vi "bigcryo_Harry-RH - step v1.vi"(6 "Mag Field Step":dbl=0.002, 7 "Directory Output":string="C:\\User Data\\hlb54\\210111_42B\\JJ1\\IcH_pos_to_neg_T=4p00K_set=0p0T", 8 "Stop Field":dbl=-0.2, 9 "Start Field (T)":dbl=0.2 format="%#_7f", 10 "Stop":bool, 11 "Measure":bool) -> ()   [LabVIEW 2019]
uses:
  Global 2.vi
  B_Globals.vi
  <vilib>/Utility/file.llb/Read From Spreadsheet File (DBL).vi
panel:
  out "B [T]":dbl
  out "Sample Temp [K] - Meas":dbl=1.55928
  out "I - Count":cluster{i32[], dbl[]}(graph) caption="XY Graph"
  out "Status":string="Welcome!"
  in  "Keithley":refnum<visa-resource-name>="GPIB1::20::INSTR"
  in  "Delay [sec]":dbl=0.002 format="%#_6e"
  in  "Compliance [V] 2":dbl=10.0 format="%#_6f"
  in  "Abort Conductance":bool
  in  "Count [A]":dbl=1e-05 format="%#_6e"
  in  "I-Max [A]":dbl=0.002 format="%#_6e"
  in  "Arm Conductance":bool
  in  "Minicryo":bool=TRUE
  in  "Field and rate":dbl[][](array[numeric])
  in  "step":bool=TRUE
  in  "Set Rate (T/min)":dbl=0.1
  out "Iteration?":i32=401
  out "B Aim":dbl=-0.202
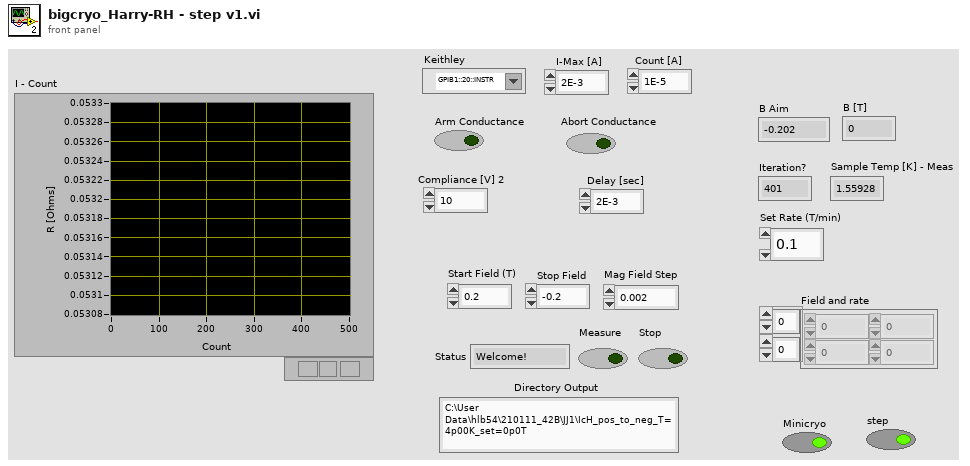
[diagram p1: front panel]
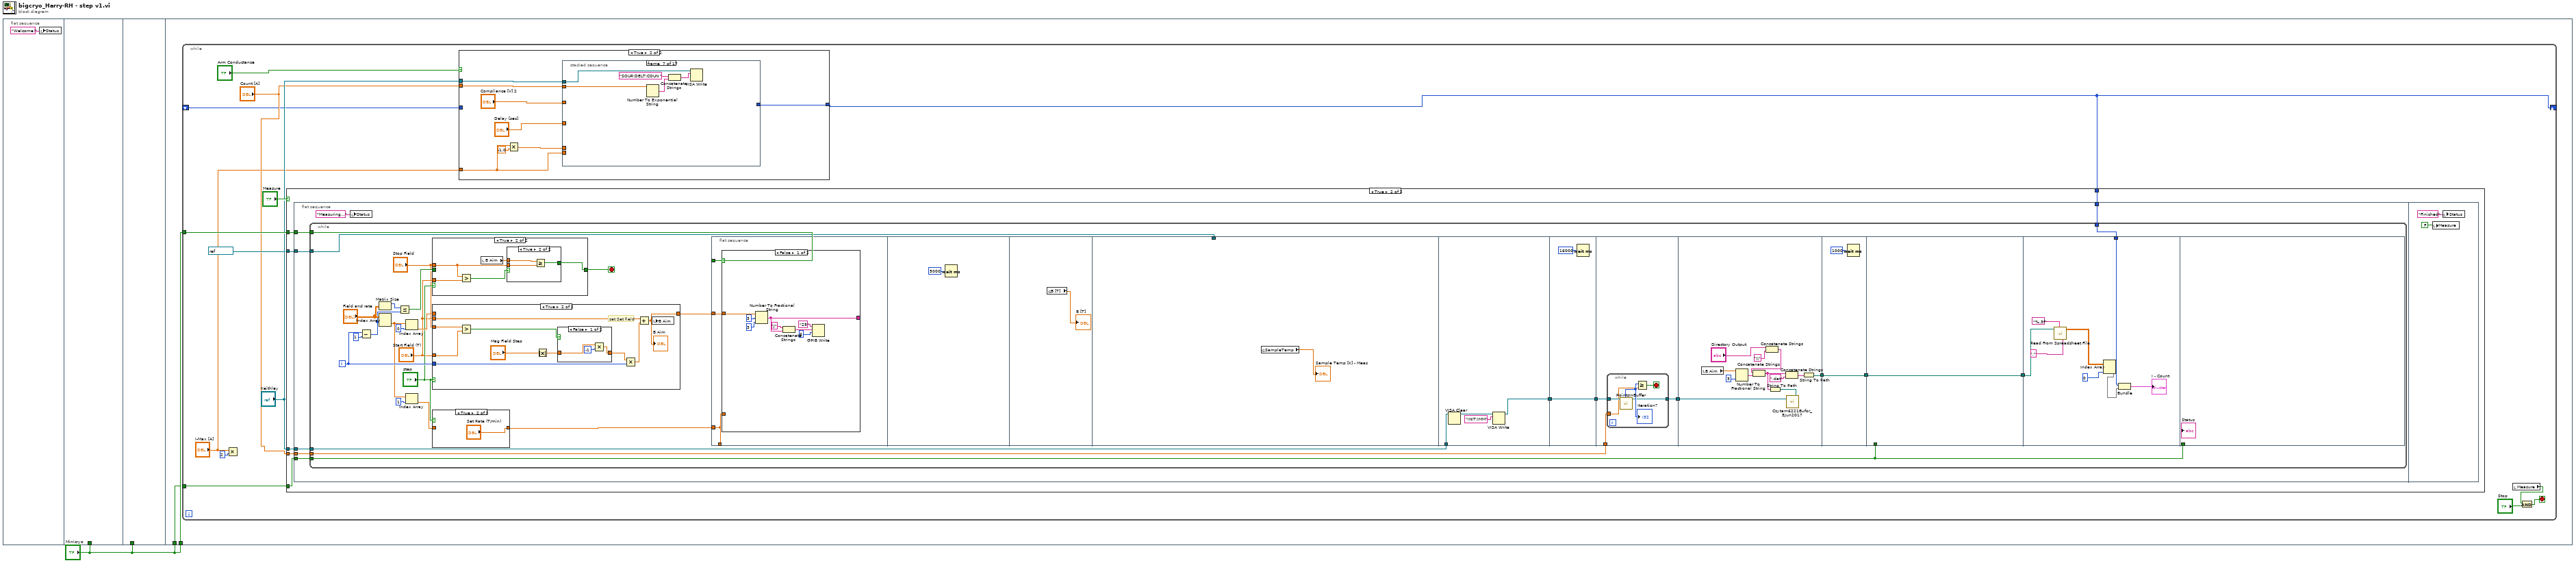
[diagram p0: block diagram]
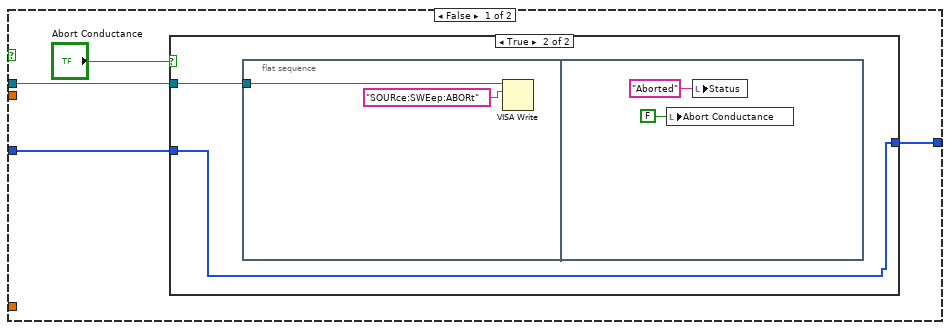
[diagram p2: hidden frame]
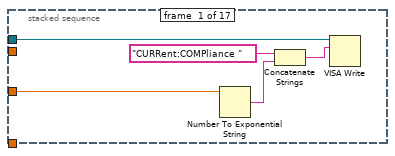
[diagram p4: hidden frame]
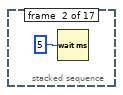
[diagram p5: hidden frame]
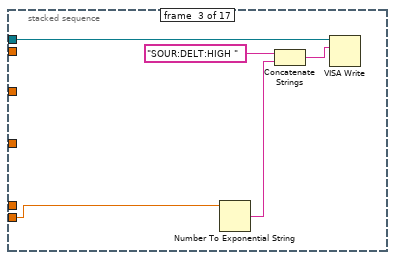
[diagram p6: hidden frame]
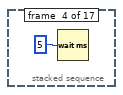
[diagram p7: hidden frame]
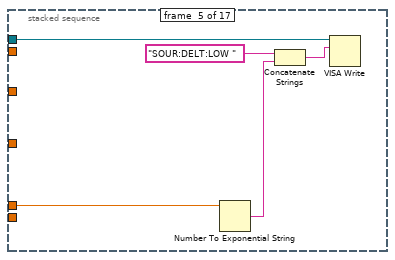
[diagram p8: hidden frame]
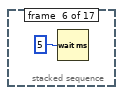
[diagram p9: hidden frame]
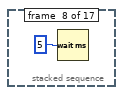
[diagram p10: hidden frame]
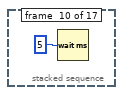
[diagram p12: hidden frame]
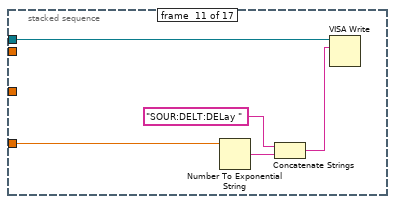
[diagram p13: hidden frame]
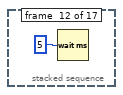
[diagram p14: hidden frame]
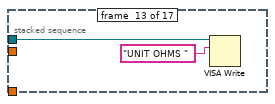
[diagram p15: hidden frame]
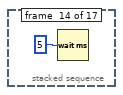
[diagram p16: hidden frame]
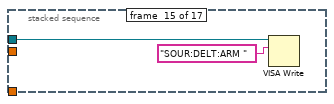
[diagram p17: hidden frame]
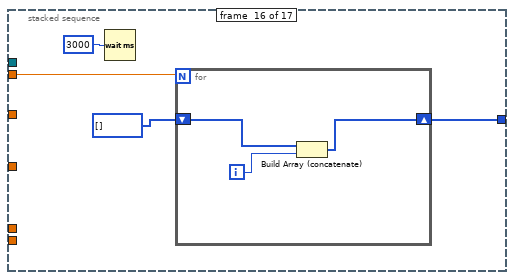
[diagram p18: hidden frame]
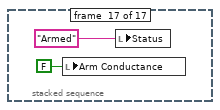
[diagram p19: hidden frame]
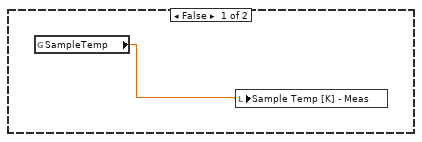
[diagram p20: hidden frame]
diagram:
  n1 = flat-sequence {
    tunnel: "Minicryo" -> [_]
    tunnel: "Minicryo" -> [_]
    tunnel: "Minicryo" -> [w4]
    tunnel: "Minicryo" -> [w3]
    frame #0 {
      n2 = local write "Status"("Welcome!") -> ()
    }
    frame #1 {
    }
    frame #2 {
    }
    frame #3 {
      n3 = while {
        tunnel: w4 -> [w18]
        tunnel: w3 -> [w17]
        shift-right: [w5] -> _
        shift-left: _ -> [w6]
        stop <- w9 stop-if-true
        n4 = Multiply(x="I-Max [A]", y=2) -> ()  [unwired: 1 out]
        n5 = case shown="True" "Arm Conductance" {
          tunnel: "Keithley" -> [w21 w34]
          tunnel: "Count [A]" -> [_ w33]
          tunnel: "I-Max [A]" -> [_ w31]
          tunnel: [w19 w30] -> w5
          tunnel: w6 -> [w20 _]
          frame False {
            n6 = case shown="True" "Abort Conductance" {
              tunnel: w21 -> [_ w25]
              tunnel: w20 -> [w23 w24]
              tunnel: [w23 w24] -> w19
              frame False {
              }
              frame True {
                n7 = flat-sequence {
                  tunnel: w25 -> [w26]
                  frame #0 {
                    n8 = VISA Write(VISA resource name=w26, write buffer="SOURce:SWEep:ABORt") -> ()  [unwired: 1 in, 3 out]
                  }
                  frame #1 {
                    n9 = local write "Abort Conductance"(FALSE) -> ()
                    n10 = local write "Status"("Aborted") -> ()
                  }
                }
              }
            }
          }
          frame True {
            n11 = Multiply(x=w31, y=-1.0) -> (x*y=w32:dbl)
            n12 = stacked-sequence {
              tunnel: w32 -> [_ _ _ _ w50 _ _ _ _ _ _ _ _ _ _ _ _]
              tunnel: "Delay [sec]" -> [_ _ _ _ _ _ _ _ _ _ w64 _ _ _ _ _ _]
              tunnel: "Compliance [V] 2" -> [w39 _ _ _ _ _ _ _ _ _ _ _ _ _ _ _ _]
              tunnel: w34 -> [w38 _ w45 _ w51 _ w57 _ _ _ w63 _ w69 _ w72 _ _]
              tunnel: w33 -> [_ _ _ _ _ _ w56 _ _ _ _ _ _ _ _ w74 _]
              tunnel: w31 -> [_ _ w44 _ _ _ _ _ _ _ _ _ _ _ _ _ _]
              tunnel: [_ _ _ _ _ _ _ _ _ _ _ _ _ _ _ w75 _] -> w30
              frame #0 {
                n13 = Number To Exponential String(number=w39) -> (E-format string=w41:string)  [unwired: 3 in]
                n14 = Concatenate Strings("CURRent:COMPliance ", w41) -> (w40:string)
                n15 = VISA Write(VISA resource name=w38, write buffer=w40) -> ()  [unwired: 1 in, 3 out]
              }
              frame #1 {
                n16 = Wait (ms)(milliseconds to wait=5) -> ()  [unwired: 1 out]
              }
              frame #2 {
                n17 = Number To Exponential String(number=w44) -> (E-format string=w47:string)  [unwired: 3 in]
                n18 = Concatenate Strings("SOUR:DELT:HIGH ", w47) -> (w46:string)
                n19 = VISA Write(VISA resource name=w45, write buffer=w46) -> ()  [unwired: 1 in, 3 out]
              }
              frame #3 {
                n20 = Wait (ms)(milliseconds to wait=5) -> ()  [unwired: 1 out]
              }
              frame #4 {
                n21 = Number To Exponential String(number=w50) -> (E-format string=w53:string)  [unwired: 3 in]
                n22 = Concatenate Strings("SOUR:DELT:LOW ", w53) -> (w52:string)
                n23 = VISA Write(VISA resource name=w51, write buffer=w52) -> ()  [unwired: 1 in, 3 out]
              }
              frame #5 {
                n24 = Wait (ms)(milliseconds to wait=5) -> ()  [unwired: 1 out]
              }
              frame #6 {
                n25 = Number To Exponential String(number=w56) -> (E-format string=w59:string)  [unwired: 3 in]
                n26 = Concatenate Strings("SOUR:DELT:COUN ", w59) -> (w58:string)
                n27 = VISA Write(VISA resource name=w57, write buffer=w58) -> ()  [unwired: 1 in, 3 out]
              }
              frame #7 {
                n28 = Wait (ms)(milliseconds to wait=5) -> ()  [unwired: 1 out]
              }
              frame #8 {
              }
              frame #9 {
                n29 = Wait (ms)(milliseconds to wait=5) -> ()  [unwired: 1 out]
              }
              frame #10 {
                n30 = Number To Exponential String(number=w64) -> (E-format string=w66:string)  [unwired: 3 in]
                n31 = Concatenate Strings("SOUR:DELT:DELay ", w66) -> (w65:string)
                n32 = VISA Write(VISA resource name=w63, write buffer=w65) -> ()  [unwired: 1 in, 3 out]
              }
              frame #11 {
                n33 = Wait (ms)(milliseconds to wait=5) -> ()  [unwired: 1 out]
              }
              frame #12 {
                n34 = VISA Write(VISA resource name=w69, write buffer="UNIT OHMS ") -> ()  [unwired: 1 in, 3 out]
              }
              frame #13 {
                n35 = Wait (ms)(milliseconds to wait=5) -> ()  [unwired: 1 out]
              }
              frame #14 {
                n36 = VISA Write(VISA resource name=w72, write buffer="SOUR:DELT:ARM ") -> ()  [unwired: 1 in, 3 out]
              }
              frame #15 {
                n37 = Wait (ms)(milliseconds to wait=3000) -> ()  [unwired: 1 out]
                n38 = for {
                  N: w74 -> [_]
                  shift-right: [w79] -> w75
                  shift-left: i32[] [] -> [w80]
                  i -> [w78]
                  n39 = Build Array (concatenate)(w80, w78) -> (w79:i32[])
                }
              }
              frame #16 {
                n40 = local write "Arm Conductance"(FALSE) -> ()
                n41 = local write "Status"("Armed") -> ()
              }
            }
          }
        }
        n42 = case shown="True" "Measure" {
          tunnel: w18 -> [_ w89]
          tunnel: w17 -> [_ w88]
          tunnel: "Keithley" -> [_ w87]
          tunnel: "Count [A]" -> [_ w86]
          tunnel: refnum<visa-resource-name> "COM7" ("LakeShore340") -> [_ w85]
          tunnel: w5 -> [_ w84]
          frame False {
            n43 = global read "Global 2.vi" "SampleTemp"() -> (w83:dbl)
            n44 = local write "Sample Temp [K] - Meas"(w83) -> ()
          }
          frame True {
            n45 = flat-sequence {
              tunnel: w89 -> [w96]
              tunnel: w88 -> [w95]
              tunnel: w87 -> [w94]
              tunnel: w86 -> [w93]
              tunnel: w85 -> [w91]
              tunnel: w84 -> [w90]
              frame #0 {
                n46 = while {
                  tunnel: w96 -> [w113]
                  tunnel: w95 -> [w108]
                  tunnel: w94 -> [w106]
                  tunnel: w93 -> [w105]
                  tunnel: w91 -> [w98]
                  tunnel: w90 -> [w97]
                  i -> [w119]
                  stop <- w104 stop-if-true
                  n47 = Subtract(x=w119, y=1) -> (x-y=w110:i32)
                  n48 = Matrix Size(0:"Field and rate") -> (1:w111:i32)  [unwired: 1 out]
                  n49 = Index Array(array="Field and rate", index (row)=w110) -> (element=w116:dbl[])  [unwired: 1 in]
                  n50 = Less Or Equal?(x=w111, y=w110) -> (x <= y?=w109:bool)
                  n51 = Index Array(array=w116, index=0) -> (element=w115:dbl)
                  n52 = Index Array(array=w116, index=1) -> (element=w114:dbl)
                  n53 = case shown="True" "step" {
                    tunnel: [w126 w131] -> w104
                    tunnel: w109 -> [w126 _]
                    tunnel: "Stop Field" -> [_ w129]
                    tunnel: "Start Field (T)" -> [_ w128]
                    frame False {
                    }
                    frame True {
                      n54 = Greater?(x=w129, y=w128) -> (0:w127:bool)
                      n55 = local read "B Aim"() -> (w130:dbl)
                      n56 = case shown="True" w127 {
                        tunnel: [w134 w137] -> w131
                        tunnel: w130 -> [w132 w136]
                        tunnel: w129 -> [w133 w135]
                        frame False {
                          n57 = Less Or Equal?(x=w132, y=w133) -> (x <= y?=w134:bool)
                        }
                        frame True {
                          n58 = Greater Or Equal?(x=w136, y=w135) -> (x >= y?=w137:bool)
                        }
                      }
                    }
                  }
                  n59 = case shown="True" "step" {
                    tunnel: [w140 w149] -> w125
                    tunnel: w119 -> [_ w148]
                    tunnel: w115 -> [w140 _]
                    tunnel: "Start Field (T)" -> [_ w147]
                    tunnel: "Start Field (T)" -> [_ w146]
                    tunnel: "Stop Field" -> [_ w145]
                    frame False {
                    }
                    frame True {
                      # "set Set field"
                      n60 = Greater?(x=w145, y=w146) -> (0:w141:bool)
                      n61 = Absolute Value(x="Mag Field Step") -> (abs(x)=w143:dbl)
                      n62 = case shown="False" w141 {
                        tunnel: [w153 w154] -> w142
                        tunnel: w143 -> [w151 w154]
                        frame False {
                          n63 = Multiply(x=w151, y=-1) -> (x*y=w153:dbl)
                        }
                        frame True {
                        }
                      }
                      n64 = Multiply(x=w142, y=w148) -> (x*y=w150:dbl)
                      n65 = Add(x=w147, y=w150) -> (x+y=w149:dbl)
                      "B Aim" <- w149
                      n66 = local write "B Aim"(w149) -> ()
                    }
                  }
                  n67 = case shown="True" "step" {
                    tunnel: [w138 "Set Rate (T/min)"] -> w121
                    tunnel: w114 -> [w138 _]
                    frame False {
                    }
                    frame True {
                    }
                  }
                  n68 = flat-sequence {
                    tunnel: w125 -> [w157]
                    tunnel: [w156] -> _
                    tunnel: w121 -> [w156]
                    tunnel: w113 -> [w155]
                    tunnel: w98 -> [_]
                    tunnel: [w176] -> w123
                    tunnel: w106 -> [w175]
                    tunnel: [w180] -> w124
                    tunnel: w123 -> [w180]
                    tunnel: w124 -> [w183]
                    tunnel: [w182] -> w122
                    tunnel: w105 -> [w181]
                    tunnel: w122 -> [w196]
                    tunnel: [w192] -> w99
                    tunnel: [w201] -> w100
                    tunnel: w99 -> [w201]
                    tunnel: w108 -> [_]
                    tunnel: [w203] -> w101
                    tunnel: w100 -> [w203]
                    tunnel: w101 -> [w209]
                    tunnel: w97 -> [w208]
                    tunnel: w108 -> [_]
                    frame #0 {
                      n69 = case shown="False" w155 {
                        tunnel: w157 -> [w160 w166]
                        tunnel: w156 -> [_ w168]
                        tunnel: [w158 w169] -> _
                        frame False {
                          n70 = Number To Fractional String(number=w160, width (-)=i16 3, precision (6)=i16 3) -> (F-format string=w158:string)  [unwired: 1 in]
                          n71 = Concatenate Strings("J" ("string"), w158) -> (w159:string)
                          n72 = GPIB Write(0:"25" ("address string"), 1:w159, 2:6) -> ()  [unwired: 2 in, 2 out]
                        }
                        frame True {
                          w167 = TRUE
                          n73 = global write "B_Globals.vi" "Remote_set"(w166) -> ()
                          n74 = global write "B_Globals.vi" "Remote_run"(w167) -> ()
                          n75 = global write "B_Globals.vi" "Remote_Rate"(w168) -> ()
                          n76 = global write "B_Globals.vi" "Remote_Go"(w167) -> ()
                          n77 = Number To Fractional String(number=w166, width (-)=i16 3, precision (6)=i16 3) -> (F-format string=w169:string)  [unwired: 1 in]
                        }
                      }
                    }
                    frame #1 {
                      n78 = Wait (ms)(milliseconds to wait=u32 5000) -> ()  [unwired: 1 out]
                    }
                    frame #2 {
                      n79 = global read "B_Globals.vi" "B [T]"() -> (→"B [T]":dbl)
                    }
                    frame #3 {
                      n80 = global read "Global 2.vi" "SampleTemp"() -> (→"Sample Temp [K] - Meas":dbl)
                    }
                    frame #4 {
                      n81 = VISA Clear(VISA resource name=w175) -> (VISA resource name out=w178:refnum<visa-resource-name>)  [unwired: 1 in, 1 out]
                      n82 = VISA Write(VISA resource name=w178, write buffer="INIT:IMM") -> (VISA resource name out=w176:refnum<visa-resource-name>)  [unwired: 1 in, 2 out]
                    }
                    frame #5 {
                      n83 = Wait (ms)(milliseconds to wait=16000) -> ()  [unwired: 1 out]
                    }
                    frame #6 {
                      n84 = while {
                        tunnel: w183 -> [w186]
                        tunnel: [w185] -> w182
                        tunnel: w181 -> [w184]
                        stop <- w187 stop-if-true
                        n85 = call "PointsInBuffer.vi"("VISA resource name"=w186) -> (3:w185:refnum<visa-resource-name>, "number"=w188:i32)  [unwired: 9 in]
                        "Iteration?" <- w188
                        n86 = Greater Or Equal?(x=w188, y=w184) -> (x >= y?=w187:bool)
                      }
                    }
                    frame #7 {
                      n87 = local read "B Aim"() -> (w197:dbl)
                      n88 = Number To Fractional String(number=w197, precision (6)=i16 3) -> (F-format string=w200:string)  [unwired: 2 in]
                      n89 = Concatenate Strings("Directory Output", "\\") -> (w189:string)
                      n90 = Concatenate Strings(w189, w200) -> (w194:string)
                      n91 = String To Path(string=w194) -> (path=w199:path)
                      n92 = Concatenate Strings(w194, ".dat") -> (w193:string)
                      n93 = call "Czytam6221Bufor_5Jun2017.vi"("file path (dialog if empty)"=w199, 3:w196) -> ()  [unwired: 1 in, 1 out]
                      n94 = String To Path(string=w193) -> (path=w192:path)
                    }
                    frame #8 {
                      n95 = Wait (ms)(milliseconds to wait=u32 1000) -> ()  [unwired: 1 out]
                    }
                    frame #9 {
                    }
                    frame #10 {
                      n96 = call-poly <vilib>:"Read From Spreadsheet File.vi"("delimiter (\\t)"="," ("delimiter (\\t)"), "format (%.3f)"="%.3f", "file path (dialog if empty)"=w209) -> ("all rows"=w205:dbl[][])  [unwired: 4 in, 4 out]
                      n97 = Index Array(array=w205, index (col)=0 ("index (row)")) -> (element=w207:dbl[])  [unwired: 1 in]
                      n98 = Bundle(w208, "all rows"=w207) -> (→"I - Count":cluster{i32[], "all rows":dbl[]})  [unwired: 1 in]
                    }
                    frame #11 {
                    }
                  }
                }
                n99 = local write "Status"("Measuring...") -> ()
              }
              frame #1 {
                n100 = local write "Measure"(FALSE) -> ()
                n101 = local write "Status"("Finished") -> ()
              }
            }
          }
        }
        n102 = local read "Measure"() -> (w10:bool)
        n103 = And(x=w10, y="Stop") -> (x .and. y?=w9:bool)
      }
    }
  }
